vi "Hide Animated Busy Icon with Message and Abort Button.vi"(2 "Already active? (F)":bool, 3 "Message":string, 7 "Target VI reference":refnum<vi>, 11 "Error In":errorcluster, 16 "Abort Button Name (Abort)":string="Abort", 17 "Animated Busy Icon Control Name (Animated Busy Icon)":string="Animated Busy Icon", 18 "Message Control Name (Message)":string="Message") -> (10 "Error Out":errorcluster)   [LabVIEW 2019]
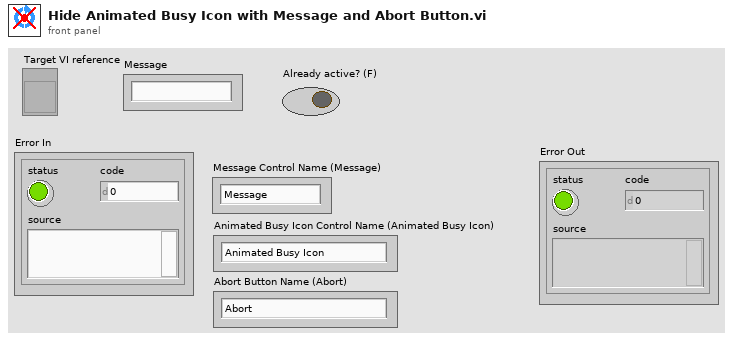
[diagram p1: front panel]
types:
  T1 = enum16{"Controls & Indicators", "Controls", "Indicators"}
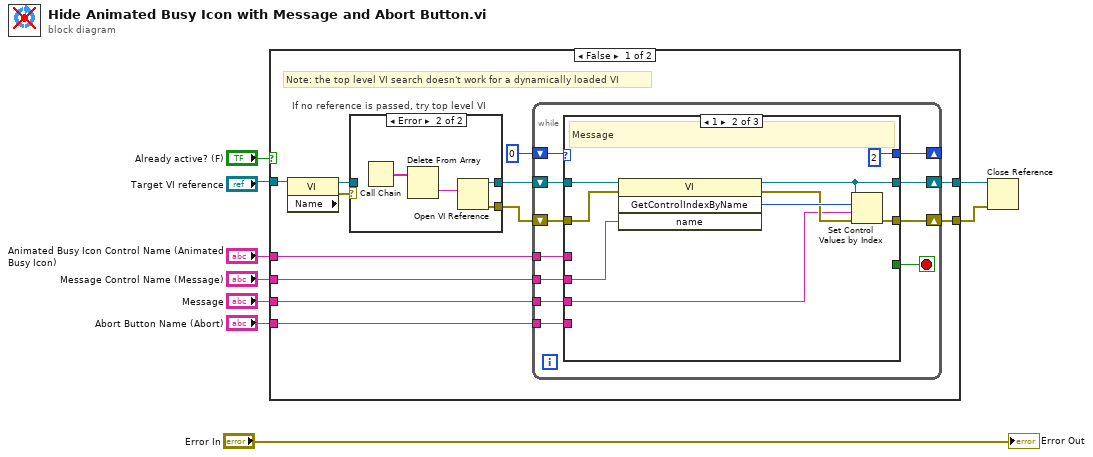
[diagram p0: block diagram]
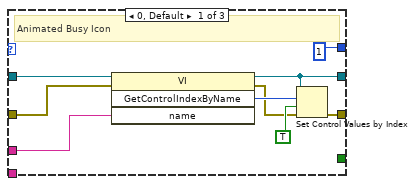
[diagram p3: hidden frame]
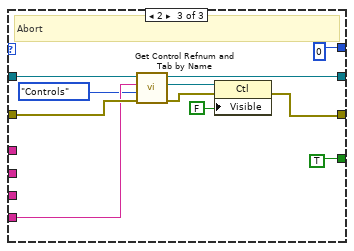
[diagram p4: hidden frame]
diagram:
  n1 = case shown="False" "Already active? (F)" {
    tunnel: [w21 w68] -> w9
    tunnel: [w20 _] -> w8
    tunnel: "Message Control Name (Message)" -> [w18 _]
    tunnel: "Animated Busy Icon Control Name (Animated Busy Icon)" -> [w17 _]
    tunnel: "Message" -> [w16 _]
    tunnel: "Target VI reference" -> [w13 w68]
    tunnel: "Abort Button Name (Abort)" -> [w10 _]
    frame False {
      # "Note: the top level VI search doesn't work for a dynamically loaded VI"
      n2 = property class="VI" props=["Name"](reference=w13) -> (reference out=w12:refnum<vi>, error out=w11:errorcluster)  [unwired: 1 in, 1 out]
      n3 = case "If no reference is passed, try top level VI" shown="Error" w11 {
        selector: w11 -> [w22 _]
        tunnel: [w22 w27] -> w14
        tunnel: [w23 w26] -> w15
        tunnel: w12 -> [w23 _]
        frame No Error {
        }
        frame Error {
          n4 = Call Chain() -> (call chain=w24:string[])
          n5 = Delete From Array(array=w24) -> (deleted portion=w25:string)  [unwired: 2 in, 1 out]
          n6 = Open VI Reference(vi path=w25) -> (vi reference=w26:refnum<vi>, error out=w27:errorcluster)  [unwired: 5 in]
        }
      }
      n7 = while {
        shift-right: [w35] -> w20
        shift-left: w14 -> [w38]
        shift-right: [w36] -> w21
        shift-left: w15 -> [w37]
        shift-right: [w33] -> _
        shift-left: 0 -> [w34]
        tunnel: w18 -> [w31]
        tunnel: w17 -> [w30]
        tunnel: w16 -> [w29]
        tunnel: w10 -> [w28]
        stop <- w32 stop-if-true
        n8 = case shown="1" w34 {
          tunnel: w38 -> [w44 w54 w62]
          tunnel: w37 -> [w43 w53 w63]
          tunnel: [w42 w52 w60] -> w36
          tunnel: [w41 w51 w58] -> w35
          tunnel: [1 2 0] -> w33
          tunnel: [_ _ TRUE] -> w32
          tunnel: w31 -> [_ w49 _]
          tunnel: w30 -> [w39 _ _]
          tunnel: w29 -> [_ w48 _]
          tunnel: w28 -> [_ _ w61]
          frame 0, Default {
            # "Animated Busy Icon"
            n9 = invoke class="VI" method="GetControlIndexByName"(reference=w43, error in=w44, "name"=w39) -> (reference out=w42:refnum<vi>, error out=w45:errorcluster, "GetControlIndexByName"=w47:i32)  [unwired: 1 in, 1 out]
            n10 = Set Control Values by Index(0:w42, 1:w47, 2:TRUE ("Visible"), 3:w45) -> (11:w41:errorcluster)
          }
          frame 1 {
            # "Message"
            n11 = invoke class="VI" method="GetControlIndexByName"(reference=w53, error in=w54, "name"=w49) -> (reference out=w52:refnum<vi>, error out=w55:errorcluster, "GetControlIndexByName"=w56:i32)  [unwired: 1 in, 1 out]
            n12 = Set Control Values by Index(0:w52, 1:w56, 2:w48, 3:w55) -> (11:w51:errorcluster)
          }
          frame 2 {
            # "Abort"
            n13 = call "Get Control Refnum and Tab by Name.vi"("error in"=w62, "Selection"=T1."Controls", "Control Label"=w61, "VI  Ref"=w63) -> ("error out"=w64:errorcluster, "Ctl Refnum"=w65:refnum<vi>, "VI  Ref (out)"=w60:refnum<vi>)  [unwired: 3 in, 2 out]
            n14 = property class="Ctl"(reference=w65, error in=w64, "Visible"=FALSE) -> (error out=w58:errorcluster)  [unwired: 1 out]
          }
        }
      }
    }
    frame True {
    }
  }
  n15 = Close Reference(reference=w9, error in (no error)=w8) -> ()  [unwired: 1 out]
  "Error Out" <- "Error In"
